vi "Process Message.vi"(8 "error in (no error)":errorcluster, 10 "Request Message":variant, 11 "GenNet Variant Protocol in":refnum<class "GenNet Variant Protocol.lvclass">) -> (0 "error out":errorcluster, 2 "Reply Message":variant, 3 "GenNet Variant Protocol out":refnum<class "GenNet Variant Protocol.lvclass">)   [LabVIEW 2020, in "hse-gennet.lvlib" / "GenNet Variant Protocol.lvclass"]
doc: "____\nHAMPEL SOFTWARE ENGINEERING v3.8.0 (2023-12-18 14:41)"
uses:
  GenNet Variant Protocol.lvclass
  C:/GitLab-Runner/builds/7NHnU7RQc/0/open-source/hse-libraries/Source/hse-gennet/GenNet Protocols/GenNet Protocol.lvclass
  GenNet Protocol.lvclass/GenNet Protocol.ctl
  <vilib>/Delacor/Delacor QMH/Libraries/Message Queue_class/Delacor_lib_QMH_Message Queue.lvclass/Delacor_lib_QMH_Message Queue.ctl
  <vilib>/Delacor/Delacor QMH/Libraries/Message Queue_class/Delacor_lib_QMH_Enqueue Message (Single).vi
  Get Notifier Timeout.vi
  Get Caller MsgQ.vi
  <vilib>/Delacor/Delacor QMH/Libraries/Message Queue_class/Delacor_lib_QMH_Message Queue.lvclass
  GenNet Variant Protocol.lvclass/GenNet Variant Protocol.ctl
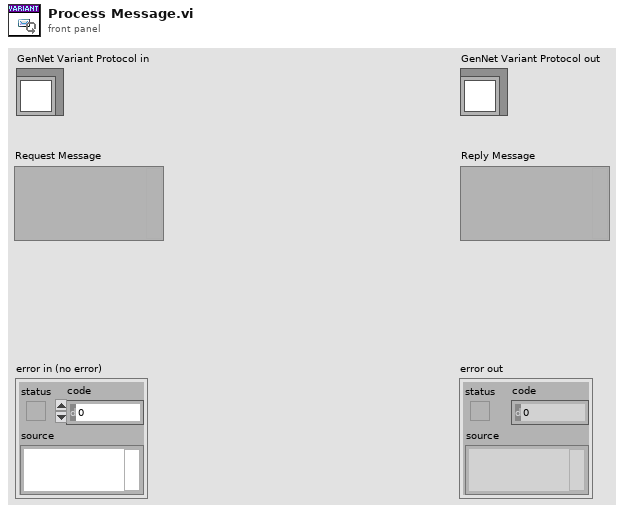
[diagram p1: front panel]
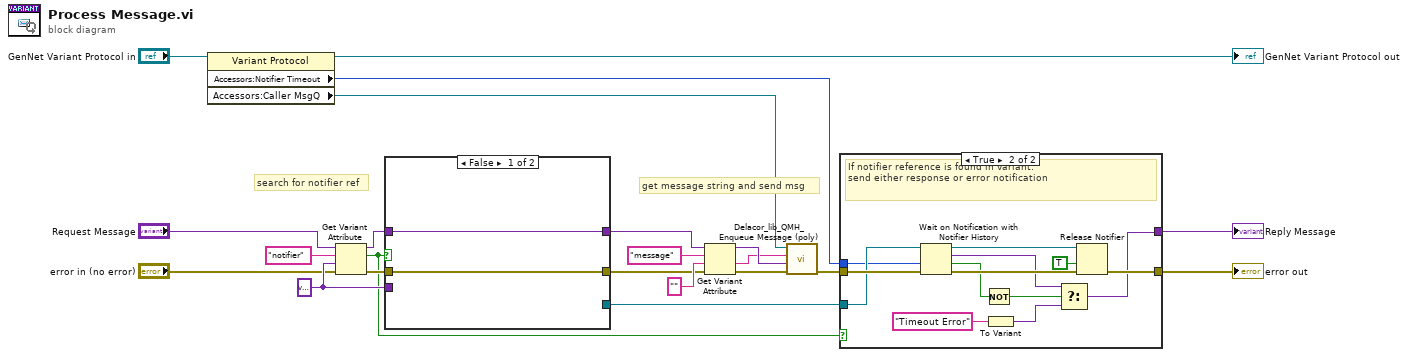
[diagram p0: block diagram]
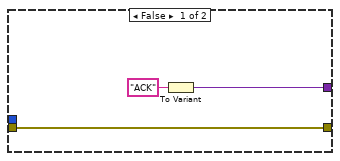
[diagram p2: hidden frame]
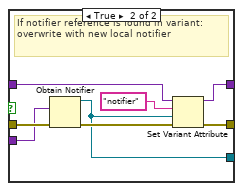
[diagram p3: hidden frame]
diagram:
  w19 = variant ("Message Data")
  # "get message string and send msg"
  # "search for notifier ref"
  n1 = property class="Variant Protocol"(reference="GenNet Variant Protocol in") -> (reference out=→"GenNet Variant Protocol out":refnum<class "GenNet Variant Protocol.lvclass">, "Accessors:Notifier Timeout"=w3:i32, "Accessors:Caller MsgQ"=w1:refnum<class "Delacor_lib_QMH_Message Queue.lvclass">)  [unwired: 1 in, 1 out]
  n2 = Get Variant Attribute(Variant="Request Message", name="notifier", default value (empty Variant)=w19, error in="error in (no error)") -> (duplicate Variant=w21:variant, found=w12:bool, error out=w20:errorcluster)  [unwired: 1 out]
  n3 = case shown="False" w12 {
    tunnel: w21 -> [w24 w29]
    tunnel: w19 -> [_ w31]
    tunnel: w20 -> [w23 w32]
    tunnel: [w24 w27] -> w15
    tunnel: [w23 w26] -> w16
    tunnel: [_ w25] -> w10
    frame False {
    }
    frame True {
      # "If notifier reference is found in variant:\noverwrite with new local notifier"
      n4 = Obtain Notifier(notification data type=w31, error in (no error)=w32) -> (notifier out=w25:refnum<notifier>, error out=w30:errorcluster)  [unwired: 2 in, 1 out]
      n5 = Set Variant Attribute(Variant=w29, name="notifier", value=w25, error in=w30) -> (Variant out=w27:variant, error out=w26:errorcluster)  [unwired: 1 out]
    }
  }
  n6 = Get Variant Attribute(Variant=w15, name="message", default value (empty Variant)="", error in=w16) -> (duplicate Variant=w14:variant, value=w9:string, error out=w13:errorcluster)  [unwired: 1 out]
  n7 = call-poly <vilib>:"Delacor_lib_QMH_Enqueue Message (poly).vi"("error in"=w13, "Message Data"=w14, "Message"=w9, "Message Queue in"=w1) -> ("error out"=w11:errorcluster)  [unwired: 6 in, 1 out]
  n8 = case shown="True" w12 {
    tunnel: w11 -> [w35 w48]
    tunnel: [w35 w44] -> w7
    tunnel: [w34 w40] -> w6
    tunnel: w10 -> [_ w47]
    tunnel: w3 -> [_ w36]
    frame False {
      n9 = To Variant(anything="ACK") -> (Variant=w34:variant)
    }
    frame True {
      # "If notifier reference is found in variant:\nsend either response or error notification"
      n10 = Wait on Notification with Notifier History(0:w47, 2:w36, 3:w48) -> (8:w46:refnum<notifier>, 9:w41:variant, 10:w42:bool, 11:w45:errorcluster)  [unwired: 1 in]
      n11 = Not(x=w42) -> (.not. x?=w37:bool)
      n12 = To Variant(anything="Timeout Error") -> (Variant=w38:variant)
      n13 = Select(t=w41, s=w37, f=w38) -> (s? t:f=w40:variant)
      n14 = Release Notifier(notifier=w46, force destroy? (F)=TRUE, error in (no error)=w45) -> (error out=w44:errorcluster)  [unwired: 2 out]
    }
  }
  "error out" <- w7
  "Reply Message" <- w6
